vi "dg535 read output.vi"(0 "GPIB address":string="15", 1 "output":u16(ring) items=["T0", "A", "B", "AB", "C", "D", "CD"], 2 "read":bool, 3 "error in":errorcluster) -> (4 "mode":u8(ring) items=["TTL", "NIM", "ECL", "VAR"], 5 "offset":dbl min=-3.0 max=4.0 format="%.2f", 6 "amplitude":dbl=1.0 min=-3.0 max=4.0 format="%.2f", 7 "inversion":bool, 8 "load":bool, 9 "error out":errorcluster)   [LabVIEW 2011]
doc: "This subVI reads the output mode, load, inversion, amplitude, and offset of one of the output BNCs . \nOUTPUT is used to specify the output BNC which is being read .\nINVERSION specifies the polarity of the logic output when TTL, NIM or ECL mode is selected .\nThe amplitude and offset set the size of the step when the output is in VARiable mode .\nLOAD configures the selected output BNC to drive either a 50 Ohm load or High Z load ."
panel:
  # "50 Ohm\nHigh Z"
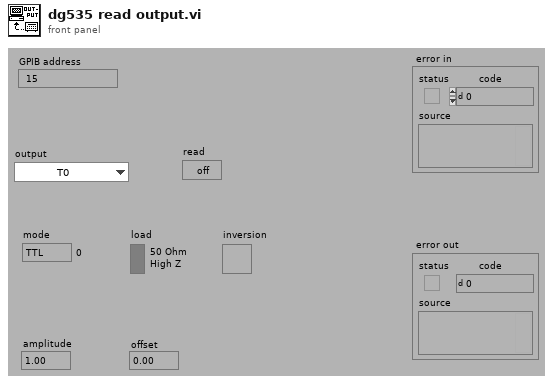
[diagram p1: front panel]
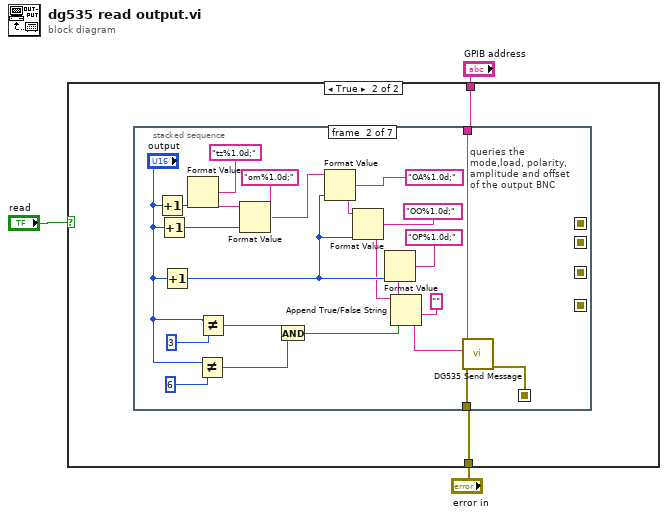
[diagram p0: block diagram]
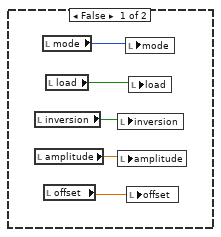
[diagram p2: hidden frame]
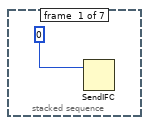
[diagram p3: hidden frame]
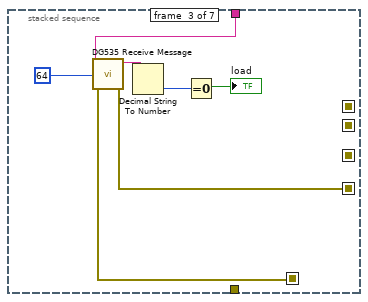
[diagram p4: hidden frame]
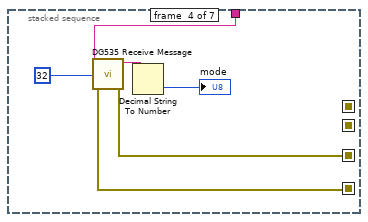
[diagram p5: hidden frame]
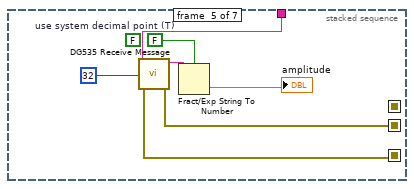
[diagram p6: hidden frame]
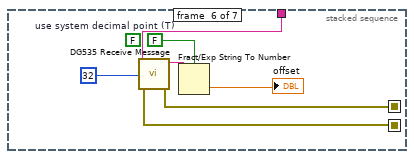
[diagram p7: hidden frame]
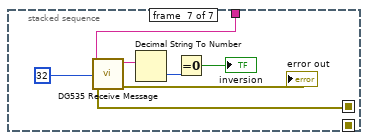
[diagram p8: hidden frame]
diagram:
  n1 = case shown="True" "read" {
    tunnel: "GPIB address" -> [_ w10]
    tunnel: "error in" -> [_ w9]
    frame False {
      n2 = local read "inversion"() -> (w6:bool)
      n3 = local read "amplitude"() -> (w5:dbl)
      n4 = local read "mode"() -> (w8:u8)
      n5 = local read "offset"() -> (w4:dbl)
      n6 = local read "load"() -> (w7:bool)
      n7 = local write "inversion"(w6) -> ()
      n8 = local write "amplitude"(w5) -> ()
      n9 = local write "mode"(w8) -> ()
      n10 = local write "offset"(w4) -> ()
      n11 = local write "load"(w7) -> ()
    }
    frame True {
      n12 = stacked-sequence {
        seq-local: [_ w18 _ _ _ _ _] -> [_ _ w37 _ _ _ _]
        seq-local: [_ _ w36 _ _ _ _] -> [_ _ _ w44 _ _ _]
        seq-local: [_ _ _ w43 _ _ _] -> [_ _ _ _ w51 _ _]
        seq-local: [_ _ _ _ w50 _ _] -> [_ _ _ _ _ w58 _]
        seq-local: [_ _ _ _ _ w57 _] -> [_ _ _ _ _ _ w64]
        tunnel: w10 -> [_ w24 w39 w46 w53 w59 w65]
        tunnel: w9 -> [_ w19 _ _ _ _ _]
        frame #0 {
          n13 = SendIFC(3:0) -> ()  [unwired: 1 in, 2 out]
        }
        frame #1 {
          # "queries the\nmode,load, polarity,\namplitude and offset\nof the output BNC"
          n14 = Increment(x="output") -> (x+1=w26:u16)
          n15 = Increment(x="output") -> (x+1=w25:u16)
          n16 = Increment(x="output") -> (x+1=w20:u16)
          n17 = Format Value(format string="tz%1.0d;", value (0)=w26) -> (output string=w17:string)  [unwired: 1 in]
          n18 = Not Equal?(x="output", y=6) -> (x != y?=w27:bool)
          n19 = Not Equal?(x="output", y=3) -> (x != y?=w23:bool)
          n20 = Format Value(string ("")=w17, format string="om%1.0d;", value (0)=w25) -> (output string=w16:string)
          n21 = And(x=w23, y=w27) -> (x .and. y?=w31:bool)
          n22 = Format Value(string ("")=w16, format string="OA%1.0d;", value (0)=w20) -> (output string=w15:string)
          n23 = Format Value(string ("")=w15, format string="OO%1.0d;", value (0)=w20) -> (output string=w13:string)
          n24 = Format Value(format string="OP%1.0d;", value (0)=w20) -> (output string=w29:string)  [unwired: 1 in]
          n25 = Append True/False String(1:w31, 2:"", 3:w29, 4:w13) -> (0:w14:string)
          n26 = call "DG535 Send Message.vi"("address string"=w24, "write buffer"=w14, "error in"=w19) -> ("error out"=w18:errorcluster)  [unwired: 4 in, 2 out]
        }
        frame #2 {
          n27 = call "DG535 Receive Message.vi"("address string"=w39, "byte count"=64, "error in"=w37) -> ("read buffer"=w41:string, "error out"=w36:errorcluster)  [unwired: 4 in, 1 out]
          n28 = Decimal String To Number(string=w41) -> (number=w40:i32)  [unwired: 2 in, 1 out]
          n29 = Equal To 0?(x=w40) -> (x = 0?=→"load":bool)
        }
        frame #3 {
          n30 = call "DG535 Receive Message.vi"("address string"=w46, "byte count"=32, "error in"=w44) -> ("read buffer"=w47:string, "error out"=w43:errorcluster)  [unwired: 4 in, 1 out]
          n31 = Decimal String To Number(string=w47) -> (number=→"mode":i32)  [unwired: 2 in, 1 out]
        }
        frame #4 {
          (unwired) FALSE ("use system decimal point (T)")
          w49 = FALSE  # use system decimal point (T)
          n32 = call "DG535 Receive Message.vi"("address string"=w53, "byte count"=32, "error in"=w51) -> ("read buffer"=w54:string, "error out"=w50:errorcluster)  [unwired: 4 in, 1 out]
          n33 = Fract/Exp String To Number(use system decimal point (T)=w49, string=w54) -> (number=→"amplitude":dbl)  [unwired: 2 in, 1 out]
        }
        frame #5 {
          (unwired) FALSE ("use system decimal point (T)")
          w56 = FALSE  # use system decimal point (T)
          n34 = call "DG535 Receive Message.vi"("address string"=w59, "byte count"=32, "error in"=w58) -> ("read buffer"=w61:string, "error out"=w57:errorcluster)  [unwired: 4 in, 1 out]
          n35 = Fract/Exp String To Number(use system decimal point (T)=w56, string=w61) -> (number=→"offset":dbl)  [unwired: 2 in, 1 out]
        }
        frame #6 {
          n36 = call "DG535 Receive Message.vi"("address string"=w65, "byte count"=32, "error in"=w64) -> ("read buffer"=w68:string, "error out"=→"error out":errorcluster)  [unwired: 4 in, 1 out]
          n37 = Decimal String To Number(string=w68) -> (number=w67:i32)  [unwired: 2 in, 1 out]
          n38 = Equal To 0?(x=w67) -> (x = 0?=→"inversion":bool)
        }
      }
    }
  }
